vi "Configure Temperature.vi"(0 "VISA resource name":refnum<visa-resource-name>, 1 "Resolution (7: 6.5 digits)":u16(ring)=7 items=["3.5 Digits"=4, "4.5 Digits"=5, "5.5 Digits"=6, "6.5 Digits"=7], 2 "Power Line Cycles (1.00)":dbl=1.0 format="%.2f", 3 "Temperature Units (0: Celsius)":u16(ring) items=["Celsius", "Fahrenheit", "Kelvin"], 5 "error in (no error)":errorcluster, 7 "Digital Filter (0: Off)":u16(ring) items=["Off", "Moving Filter", "Repeating Filter"], 9 "Digital Filter Readings (10)":i32=10, 10 "Reference (0: Off)":u16(ring) items=["Off", "Set", "Acquire"], 12 "Reference Value (0.000)":dbl format="%_3g") -> (14 "VISA resource name out":refnum<visa-resource-name>, 19 "error out":errorcluster)   [LabVIEW 2009, in "Keithley 2000.lvlib"]
doc: "This VI configures the instrument to measure temperature.\n\nNotes:\n(1) - Use the Configure Thermocouple VI to configure the thermocouple type and settings.\n(2) - Use the Configure Units VI to set the temperature units.\n(3) - When reading measurements (using the \"Data Read Single\" or \"Data Read Multiple\" VIs), a value of 9.9E+37 indicates overflow (i.e., an open circuit). Any other value is the actual temperature."
uses:
  <instrlib>/Keithley 2000/Keithley 2000.lvlib
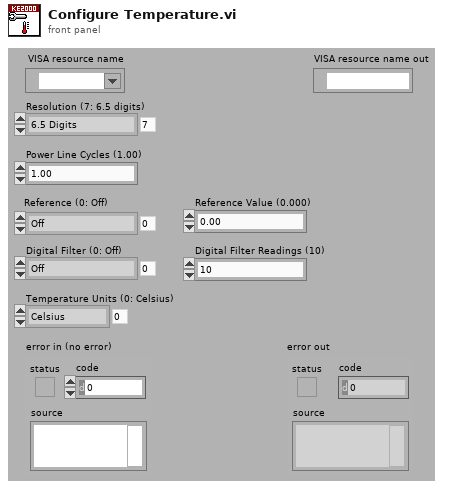
[diagram p1: front panel]
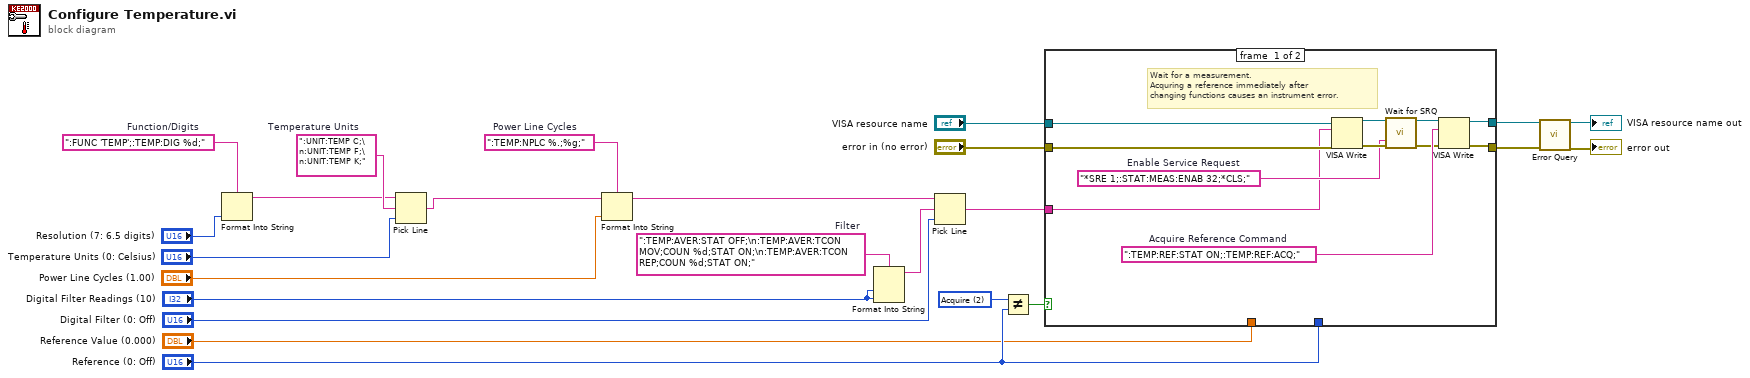
[diagram p0: block diagram]
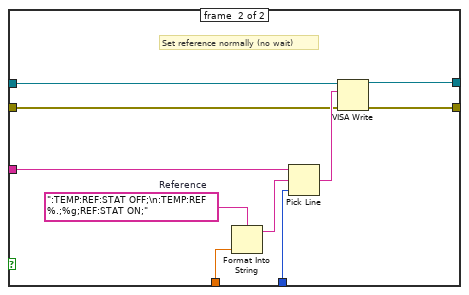
[diagram p2: hidden frame]
diagram:
  w4 = ":UNIT:TEMP C;\n:UNIT:TEMP F;\n:UNIT:TEMP K;"  # Temperature Units
  w13 = u16 2 items=["Off", "Set", "Acquire"] ("Reference (0: Off)")
  w17 = ":TEMP:NPLC %.;%g;"  # Power Line Cycles
  w19 = ":TEMP:AVER:STAT OFF;\n:TEMP:AVER:TCON MOV;COUN %d;STAT ON;\n:TEMP:AVER:TCON REP;COUN %d;STAT ON;"  # Filter
  w21 = ":FUNC 'TEMP';:TEMP:DIG %d;"  # Function/Digits
  n1 = Format Into String(format string=w21, "Resolution (7: 6.5 digits)") -> (resulting string=w3:string)  [unwired: 2 in, 1 out]
  n2 = Pick Line(string ("")=w3, multi-line string=w4, line index="Temperature Units (0: Celsius)") -> (output string=w2:string)
  n3 = Format Into String(format string=w17, initial string=w2, "Power Line Cycles (1.00)") -> (resulting string=w14:string)  [unwired: 1 in, 1 out]
  n4 = Format Into String(format string=w19, "Digital Filter Readings (10)", "Digital Filter Readings (10)") -> (resulting string=w20:string)  [unwired: 2 in, 1 out]
  n5 = Pick Line(string ("")=w14, multi-line string=w20, line index="Digital Filter (0: Off)") -> (output string=w10:string)
  n6 = Not Equal?(x=w13, y="Reference (0: Off)") -> (x != y?=w7:bool)
  n7 = case shown="False" w7 {
    tunnel: "VISA resource name" -> [w32 w38]
    tunnel: "error in (no error)" -> [w33 w37]
    tunnel: "Reference Value (0.000)" -> [_ w43]
    tunnel: w10 -> [w25 w36]
    tunnel: [w27 w42] -> w8
    tunnel: [w28 w41] -> w9
    tunnel: "Reference (0: Off)" -> [_ w39]
    frame #0 {
      w26 = "*SRE 1;:STAT:MEAS:ENAB 32;*CLS;"  # Enable Service Request
      w31 = ":TEMP:REF:STAT ON;:TEMP:REF:ACQ;"  # Acquire Reference Command
      # "Wait for a measurement.\nAcquring a reference immediately after\nchanging functions causes an instrument error."
      n8 = VISA Write(VISA resource name=w32, write buffer=w25, error in (no error)=w33) -> (VISA resource name out=w35:refnum<visa-resource-name>, error out=w34:errorcluster)  [unwired: 1 out]
      n9 = call <instrlib>:"Wait for SRQ.vi"("VISA resource name"=w35, "SRQ Enable Command"=w26, "error in (no error)"=w34) -> ("VISA resource name out"=w30:refnum<visa-resource-name>, "error out"=w29:errorcluster)  [unwired: 15 in]
      n10 = VISA Write(VISA resource name=w30, write buffer=w31, error in (no error)=w29) -> (VISA resource name out=w28:refnum<visa-resource-name>, error out=w27:errorcluster)  [unwired: 1 out]
    }
    frame #1 {
      w45 = ":TEMP:REF:STAT OFF;\n:TEMP:REF %.;%g;REF:STAT ON;"  # Reference
      # "Set reference normally (no wait)"
      n11 = Format Into String(format string=w45, w43) -> (resulting string=w44:string)  [unwired: 2 in, 1 out]
      n12 = Pick Line(string ("")=w36, multi-line string=w44, line index=w39) -> (output string=w40:string)
      n13 = VISA Write(VISA resource name=w38, write buffer=w40, error in (no error)=w37) -> (VISA resource name out=w41:refnum<visa-resource-name>, error out=w42:errorcluster)  [unwired: 1 out]
    }
  }
  n14 = call <instrlib>:"Error Query.vi"("VISA resource name"=w9, "error in (no error)"=w8) -> ("VISA resource name out"=→"VISA resource name out":refnum<visa-resource-name>, "error out"=→"error out":errorcluster)  [unwired: 14 in, 2 out]
